vi "CalculoOndaSenoide.vi"(9 "Taxa":dbl, 10 "InfoInSenoide":T1, 11 "GraphSenoide":cluster{"X":dbl, "Y":dbl}[](array[cluster])) -> (3 "XY Graph":cluster{"X":dbl, "Y":dbl}[](graph))   [LabVIEW 2019]
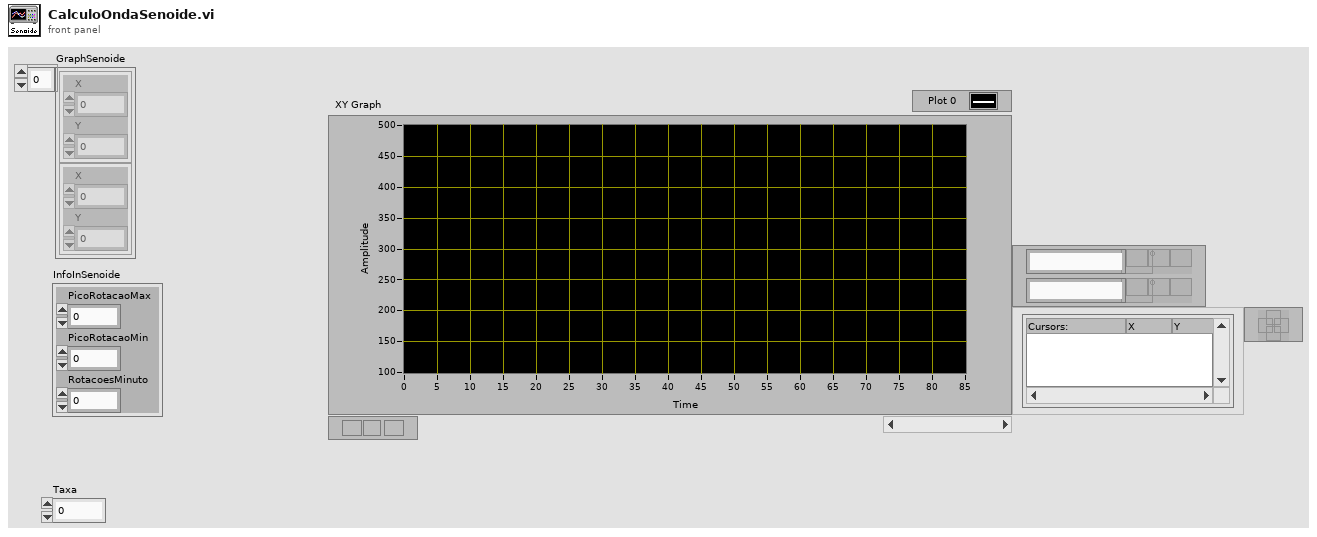
[diagram p1: front panel]
types:
  T1 = cluster{"PicoRotacaoMax":dbl, "PicoRotacaoMin":dbl, "RotacoesMinuto":dbl}
  T2 = cluster{"RotaçãoPorSeg":dbl, "Fase":dbl, "AmplitudeOnda":dbl, "Offset":dbl}
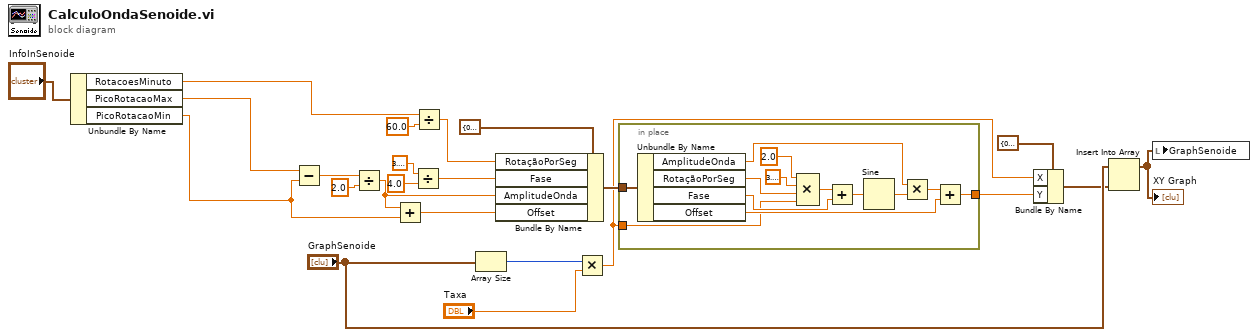
[diagram p0: block diagram]
diagram:
  n1 = Unbundle By Name("InfoInSenoide") -> ("RotacoesMinuto"=w3:dbl, "PicoRotacaoMax"=w2:dbl, "PicoRotacaoMin"=w1:dbl)
  n2 = Subtract(x=w2, y=w1) -> (x-y=w19:dbl)
  n3 = Divide(x=w19, y=2.0) -> (x/y=w15:dbl)
  n4 = Add(x=w15, y=w1) -> (x+y=w13:dbl)
  n5 = Divide(x=3.141592653589793, y=4.0) -> (x/y=w16:dbl)
  n6 = Divide(x=w3, y=60.0) -> (x/y=w17:dbl)
  n7 = Array Size(array="GraphSenoide") -> (size(s)=w6:i32)
  n8 = Bundle By Name(cluster=T2 {"RotaçãoPorSeg"=0.0, "Fase"=0.0, "AmplitudeOnda"=0.0, "Offset"=0.0}, "RotaçãoPorSeg"=w17, "Fase"=w16, "AmplitudeOnda"=w15, "Offset"=w13) -> (w14:T2)
  n9 = Multiply(x=w6, y="Taxa") -> (x*y=w5:dbl)
  n10 = in-place {
    in-place-border: [w30] -> w7
    in-place-border: w14 -> [w29]
    in-place-border: w5 -> [w24]
    n11 = Unbundle By Name(w29) -> ("AmplitudeOnda"=w26:dbl, "RotaçãoPorSeg"=w28:dbl, "Fase"=w27:dbl, "Offset"=w25:dbl)
    n12 = Compound Arithmetic op=MULTIPLY(2.0, 3.141592653589793, w28, w24) -> (w33:dbl)
    n13 = Add(x=w33, y=w27) -> (x+y=w32:dbl)
    n14 = Sine(x=w32) -> (sin(x)=w34:dbl)
    n15 = Multiply(x=w26, y=w34) -> (x*y=w31:dbl)
    n16 = Add(x=w31, y=w25) -> (x+y=w30:dbl)
  }
  n17 = Bundle By Name(cluster=cluster{"X":dbl, "Y":dbl} {"X"=0.0, "Y"=0.0} ("new element/subarray"), "X"=w5, "Y"=w7) -> (w8:cluster{"X":dbl, "Y":dbl})
  n18 = Insert Into Array(array="GraphSenoide", new element=w8) -> (w10:cluster{"X":dbl, "Y":dbl}[])  [unwired: 1 in]
  "XY Graph" <- w10
  n19 = local write "GraphSenoide"(w10) -> ()
